vi "Get All Entries.vi"(8 "error in (no error)":errorcluster, 11 "Registry in":refnum<class "Registry.lvclass">) -> (0 "error out":errorcluster, 1 "Values":variant[](array[variant]), 2 "Keys":string[](array[string]) caption="Names")   [LabVIEW 2020, in "BCI-1553 API.lvlib" / "Registry.lvlib" / "Registry.lvclass"]
doc: "Retrieves all the Key/Value pairs sotred in the registry. Does not recurse through nested Registries."
uses:
  Registry.lvclass
  Registry.lvclass/Registry.ctl
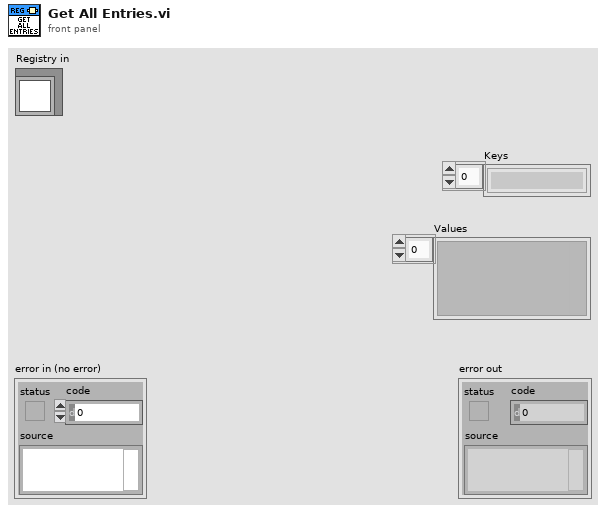
[diagram p1: front panel]
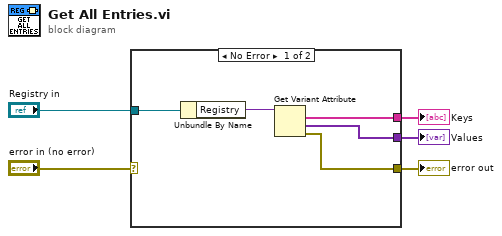
[diagram p0: block diagram]
diagram:
  n1 = case shown="No Error" "error in (no error)" {
    selector: "error in (no error)" -> [_ w11]
    tunnel: [w6 w11] -> w4
    tunnel: "Registry in" -> [w10 _]
    tunnel: [w9 _] -> w2
    tunnel: [w8 _] -> w1
    frame No Error {
      n2 = Unbundle By Name(w10) -> ("Registry"=w7:variant)
      n3 = Get Variant Attribute(Variant=w7) -> (names=w9:string[], values=w8:variant[], error out=w6:errorcluster)  [unwired: 3 in, 1 out]
    }
    frame Error {
    }
  }
  "error out" <- w4
  "Keys" <- w2
  "Values" <- w1
